vi "Read Multiple Waveforms.vi"(8 "error in (no error)":errorcluster, 9 "Timeout (10000 ms)":u32=10000, 10 "Channels":u16[](array[ring])=[0, 1] items=["Channel 1", "Channel 2", "Channel 3", "Channel 4"], 11 "VISA resource name":refnum<visa-resource-name>) -> (0 "error out":errorcluster, 2 "Waveform Data":waveform(dbl)[](graph), 3 "VISA resource name out":refnum<visa-resource-name>)   [LabVIEW 2021, in "Agilent 6000 Series.lvlib"]
doc: "Initiates an acquisition on all channels that you enabled with the <B>Configure Channel</B> VI. The VI waits for the acquisition to complete and returns the waveform for the Source Channels you specified. If the oscilloscope did not complete the acquisition within the time period you specify with the Timeout parameter, the VI returns a time out error. A common cause for a timeout error is the acquisition was not triggered. For example, the trigger level is out of range of the waveform. \n\nNote: If your instrument does not support auto compensation for probe attenuation, you may need to adjust the scaling of the Waveform Data accordingly. This is handled automatically in the <B>Configure Channel</B> VI or can be done manually by multiplying the Waveform Data by the probe attenuation."
uses:
  Agilent 6000 Series.lvlib
  Low Data VIs/Fetch Analog Waveform.vi
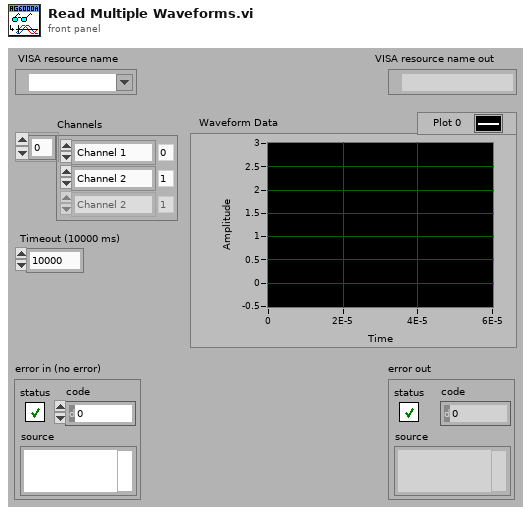
[diagram p1: front panel]
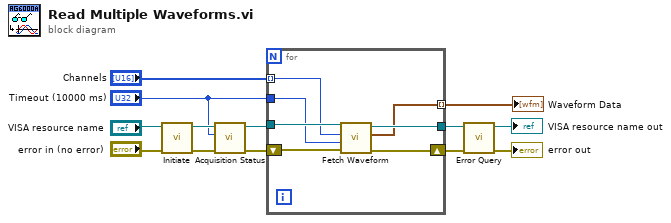
[diagram p0: block diagram]
diagram:
  n1 = call "Initiate.vi"("error in (no error)"="error in (no error)", "VISA resource name"="VISA resource name") -> ("error out"=w5:errorcluster, "VISA resource name out"=w2:refnum<visa-resource-name>)  [unwired: 8 in]
  n2 = call "Acquisition Status.vi"("error in (no error)"=w5, "Timeout (10000 ms)"="Timeout (10000 ms)", "VISA resource name"=w2) -> ("error out"=w4:errorcluster, "VISA resource name out"=w3:refnum<visa-resource-name>)  [unwired: 6 in, 1 out]
  n3 = for {
    tunnel: [w20] -> w11
    tunnel: w3 -> [w18]
    shift-right: [w19] -> w10
    shift-left: w4 -> [w17]
    tunnel: "Channels" -> [w16] mode=indexing
    tunnel: [w15] -> w6 mode=indexing
    tunnel: "Timeout (10000 ms)" -> [w14]
    n4 = call-poly "Fetch Waveform.vi"("error in (no error)"=w17, "Timeout (10000 ms)"=w14, "Source (0: Channel 1)"=w16, "VISA resource name"=w18) -> ("error out"=w19:errorcluster, "Waveform Data"=w15:waveform(dbl), "VISA resource name out"=w20:refnum<visa-resource-name>)  [unwired: 5 in]
  }
  "Waveform Data" <- w6
  n5 = call "Error Query.vi"("error in (no error)"=w10, "VISA resource name"=w11) -> ("error out"=→"error out":errorcluster, "VISA resource name out"=→"VISA resource name out":refnum<visa-resource-name>)  [unwired: 6 in, 2 out]
